vi "DAC Run.vi"(8 "error in":errorcluster, 11 "DAC Keller Diff P 23X in":refnum<class "DAC Keller Diff P 23X.lvclass">) -> (0 "error out":errorcluster, 3 "DAC Keller Diff P 23X out":refnum<class "DAC Keller Diff P 23X.lvclass">)   [LabVIEW 2019, in "DAC.lvlib" / "DAC Keller Diff P 23X.lvclass"]
uses:
  DAC Keller Diff P 23X.lvclass
  C:/Users/wg/Documents/LV_Projects/test-stand/App/DAC/DAC.lvclass
  DAC.lvclass/DAC.ctl
  Results/Results Method.ctl
  Results/DeepU Results/DeepU Results.lvclass
  DAC Keller Diff P 23X.lvclass/DAC Keller Diff P 23X.ctl
  <instrlib>/_KELLER RS485 Library/Public/Type Definitions/Channel.ctl
  DAC.lvclass
  Results/Results.lvlib
  <instrlib>/_KELLER RS485 Library/KELLER RS485 Library.lvlib
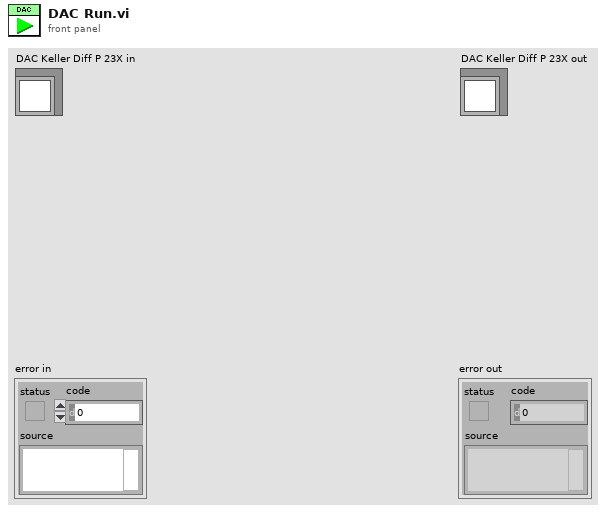
[diagram p1: front panel]
types:
  T1 = typedef "Results.lvlib/Results Method.ctl" = enum16{"Get", "Set"}
  T2 = typedef "KELLER RS485 Library.lvlib/Channel.ctl" = enum16{"CH0", "P1", "P2", "T", "TOB1", "TOB2", "TE", "CH7", "CH8", "CH9", "ConTc", "ConRaw", "CH12"}
  T3 = typedef "KELLER RS485 Library.lvlib/Bus.ctl" = cluster{"VISA":refnum<visa-resource-name>, "Baud Rate ":T4, "Timeout":u32, "Echo?":bool, "Wait before transmit":u32}
  T4 = typedef "KELLER RS485 Library.lvlib/Baud Rate.ctl" = enum16{"9600bd", "115200bd"}
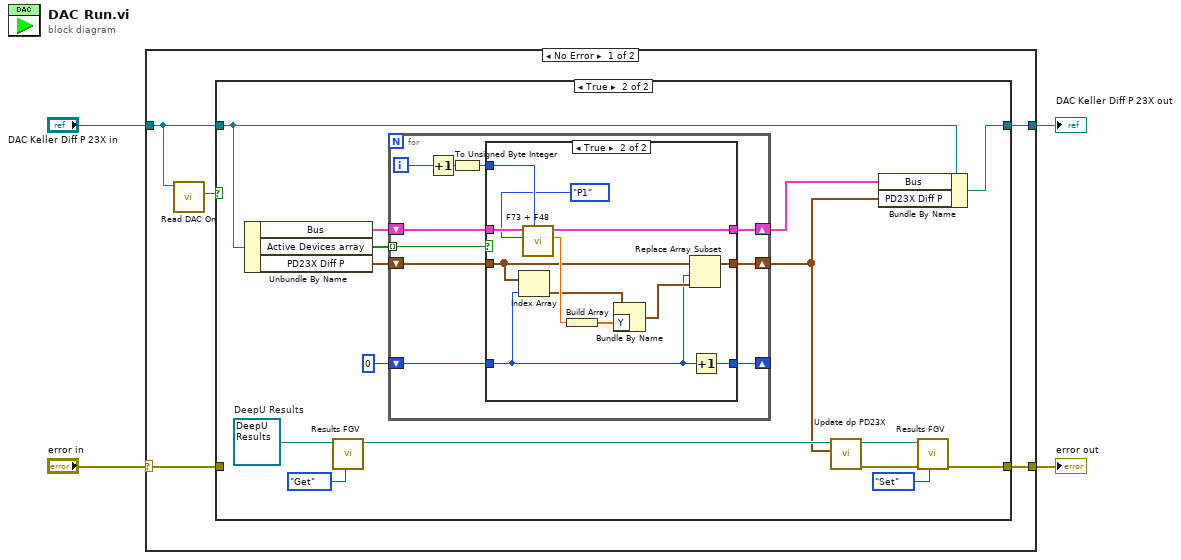
[diagram p0: block diagram]
diagram:
  n1 = case shown="No Error" "error in" {
    selector: "error in" -> [w7 w53]
    tunnel: [w6 w53] -> w2
    tunnel: [w8 w52] -> w1
    tunnel: "DAC Keller Diff P 23X in" -> [w5 w52]
    frame No Error {
      n2 = call "Read DAC On.vi"("DAC in"=w5) -> ("DAC On"=w9:bool)  [unwired: 8 in, 2 out]
      n3 = case shown="True" w9 {
        tunnel: w5 -> [w11 w26]
        tunnel: [w11 w18] -> w8
        tunnel: w7 -> [w10 _]
        tunnel: [w10 w22] -> w6
        frame False {
        }
        frame True {
          w25 = refnum<class "DeepU Results.lvclass"> refnum  # DeepU Results
          n4 = Unbundle By Name(w26) -> ("Bus"=w17:T3, "Active Devices array"=w16:bool[], "PD23X Diff P"=w15:waveform(sgl)[])
          n5 = call-dynamic "Results FGV.vi"("Method"=Results_Method."Get", "DeepU Results in"=w25) -> ("DeepU Results out"=w20:refnum<class "DeepU Results.lvclass">)  [unwired: 8 in, 1 out]
          n6 = for {
            tunnel: w16 -> [w33] mode=indexing
            shift-right: [w31] -> w12
            shift-left: w15 -> [w32]
            shift-right: [w30] -> w14
            shift-left: w17 -> [w35]
            shift-right: [w27] -> _
            shift-left: 0 -> [w28]
            i -> [w29]
            n7 = Increment(x=w29) -> (x+1=w36:i32)
            n8 = To Unsigned Byte Integer(number=w36) -> (unsigned 8bit integer=w34:u8)
            n9 = case shown="True" w33 {
              tunnel: w35 -> [w38 w51]
              tunnel: w34 -> [_ w50]
              tunnel: w32 -> [w39 w42]
              tunnel: [w39 w49] -> w31
              tunnel: [w38 w48] -> w30
              tunnel: w28 -> [w37 w40]
              tunnel: [w37 w43] -> w27
              frame False {
              }
              frame True {
                n10 = Index Array(array=w42, index=w40) -> (element=w41:waveform(sgl))
                n11 = call <instrlib>:"F73 + F48.vi"("Address (250)"=w50, "Channel (P1)"=Channel."P1", "Bus in"=w51) -> ("Value as Single"=w46:sgl, "Bus out"=w48:T3)  [unwired: 4 in, 3 out]
                n12 = Build Array(w46) -> (w45:sgl[])
                n13 = Bundle By Name(cluster=w41, "Y"=w45) -> (w44:waveform(sgl))
                n14 = Replace Array Subset(array=w42, new element=w44, index=w40) -> (w49:waveform(sgl)[])
                n15 = Increment(x=w40) -> (x+1=w43:i32)
              }
            }
          }
          n16 = call "Update dp PD23X.vi"("dp PD-23X"=w12, "DeepU Results in"=w20) -> ("error out"=w21:errorcluster, "DeepU Results out"=w19:refnum<class "DeepU Results.lvclass">)  [unwired: 8 in]
          n17 = Bundle By Name(cluster=w26, "Bus"=w14, "PD23X Diff P"=w12) -> (w18:refnum<class "DAC Keller Diff P 23X.lvclass">)
          n18 = call-dynamic "Results FGV.vi"("Method"=Results_Method."Set", "error in"=w21, "DeepU Results in"=w19) -> ("error out"=w22:errorcluster)  [unwired: 7 in, 1 out]
        }
      }
    }
    frame Error {
    }
  }
  "error out" <- w2
  "DAC Keller Diff P 23X out" <- w1
